vi "Multi-Tone Simulator.vi"() -> ()   [LabVIEW 2016]
uses:
  <vilib>/Analysis/5stat.llb/RMS (DBL).vi
  <vilib>/Analysis/NI_AALBase.lvlib
  <vilib>/Analysis/NI_AALPro.lvlib
panel:
  in  "dt":dbl=20480.0 format="%#_13g"
  in  "deltaF":i32=5
  in  "Start freq.":i32
  in  "Amplitude":dbl=0.1 format="%#_13g"
  in  "#Sample":i32=40960
  in  "#Freq.":i32=10
  out "Simulated waveform":waveform(dbl)(graph) caption="출력 웨이브폼"
  out "Crest ratio":dbl
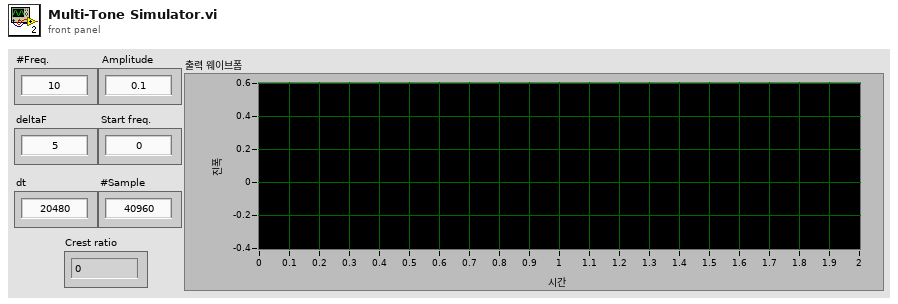
[diagram p1: front panel]
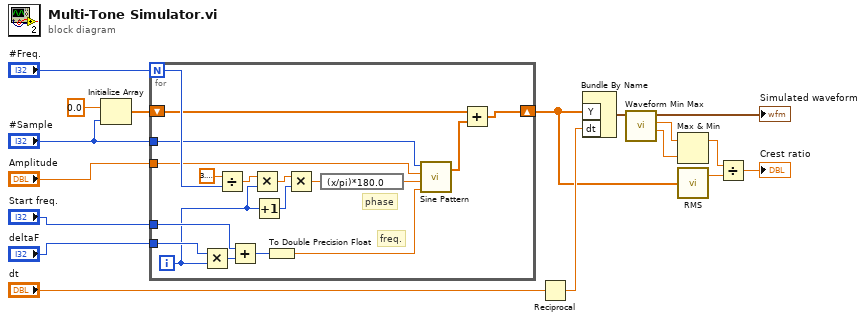
[diagram p0: block diagram]
diagram:
  n1 = Initialize Array(0.0 ("원소"), "#Sample") -> (w11:dbl[])
  n2 = for {
    N: "#Freq." -> [w29]
    tunnel: "deltaF" -> [w35]
    tunnel: "Start freq." -> [w32]
    tunnel: "#Sample" -> [w22]
    tunnel: "Amplitude" -> [w21]
    shift-right: [w20] -> w3
    shift-left: w11 -> [w19]
    i -> [w26]
    # "phase"
    # "freq."
    n3 = Multiply(x=w35, y=w26) -> (x*y=w34:i32)
    n4 = Divide(x=3.141592653589793, y=w29) -> (x/y=w31:dbl)
    n5 = Add(x=w32, y=w34) -> (x+y=w33:i32)
    n6 = Multiply(x=w31, y=w26) -> (x*y=w28:dbl)
    n7 = Increment(x=w26) -> (x+1=w27:i32)
    n8 = To Double Precision Float(number=w33) -> (double precision float=w23:dbl)
    n9 = Multiply(x=w28, y=w27) -> (x*y=w25:dbl)
    n10 = expression code="(x/pi)*180.0" ("라디안을 도로")(w25) -> (w24:dbl)
    n11 = call <vilib>:"Sine Pattern.vi"("cycles"=w23, "phase(degrees)"=w24, "amplitude"=w21, "samples"=w22) -> ("Sinusoidal Pattern"=w18:dbl[])  [unwired: 1 out]
    n12 = Add(x=w19, y=w18) -> (x+y=w20:dbl[])
  }
  n13 = Reciprocal(x="dt") -> (1/x=w10:dbl)
  n14 = Bundle By Name("Y"=w3, "dt"=w10) -> (w2:waveform(dbl))  [unwired: 1 in]
  n15 = call <vilib>:"Waveform Min Max.vi"("waveform in"=w2) -> ("Y min"=w7:dbl, "Y max"=w8:dbl, "waveform out"=→"Simulated waveform":waveform(dbl))  [unwired: 5 in, 3 out]
  n16 = Max & Min(x=w8, y=w7) -> (max(x,y)=w6:dbl)  [unwired: 1 out]
  n17 = call-poly <vilib>:"RMS.vi"("X"=w3) -> ("rms value"=w5:dbl)  [unwired: 1 out]
  n18 = Divide(x=w6, y=w5) -> (x/y=→"Crest ratio":dbl)
